vi "OAT State Machine Generate Events for Strings.vi"(1 "Initialize":bool, 2 "Strings":string[](array[string]), 4 "Event":enum16{"Changed"}[](array[ring])) -> (7 "Event Found?":bool[](array[boolean]))   [LabVIEW 2017]
doc: "Detects events for the String objects. When the string is changed, the output is set as TRUE."
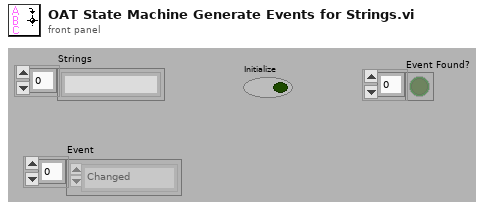
[diagram p1: front panel]
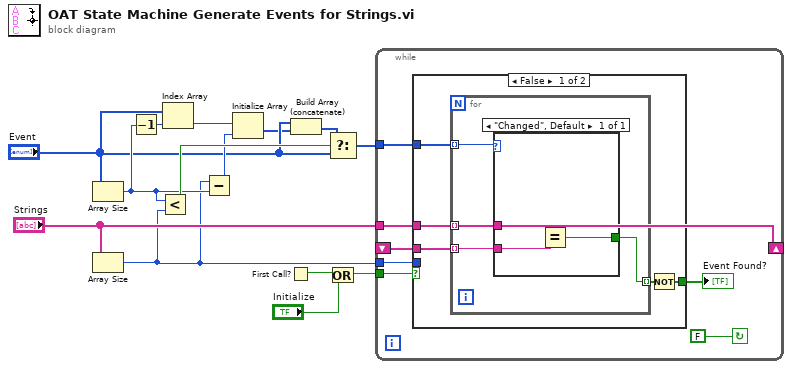
[diagram p0: block diagram]
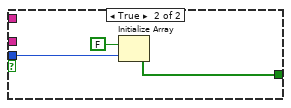
[diagram p2: hidden frame]
diagram:
  n1 = Array Size(array="Event") -> (size(s)=w9:i32)
  n2 = Array Size(array="Strings") -> (size(s)=w4:i32)
  n3 = Decrement(x=w9) -> (x-1=w10:i32)
  n4 = Less?(x=w9, y=w4) -> (x < y?=w11:bool)
  n5 = Index Array(array="Event", index=w10) -> (element=w13:enum16{"Changed"})
  n6 = Subtract(x=w4, y=w9) -> (x-y=w8:i32)
  n7 = Initialize Array(w13, w8) -> (w5:enum16{"Changed"}[])
  n8 = First Call?() -> (First Call?: T/F=w3:bool)
  n9 = Build Array (concatenate)("Event", w5) -> (w7:enum16{"Changed"}[])
  n10 = Select(t=w7, s=w11, f="Event") -> (s? t:f=w12:enum16{"Changed"}[])
  n11 = Or(x=w3, y="Initialize") -> (x .or. y?=w1:bool)
  n12 = while {
    tunnel: w4 -> [w15]
    tunnel: w1 -> [w16]
    tunnel: "Strings" -> [w19]
    shift-left: _ -> [w20]
    shift-right: [w19] -> _
    tunnel: w12 -> [w21]
    stop <- FALSE continue-if-true
    n13 = case shown="False" w16 {
      tunnel: w21 -> [w26 _]
      tunnel: w20 -> [w25 _]
      tunnel: w19 -> [w24 _]
      tunnel: [w22 w34] -> w17
      tunnel: w15 -> [_ w36]
      frame False {
        n14 = for {
          tunnel: w26 -> [w30] mode=indexing
          tunnel: w25 -> [w28] mode=indexing
          tunnel: w24 -> [w29] mode=indexing
          tunnel: [w27] -> w23 mode=indexing
          n15 = case shown="\"Changed\", Default" w30 {
            tunnel: w29 -> [w33]
            tunnel: w28 -> [w32]
            tunnel: [w31] -> w27
            frame "Changed", Default {
              n16 = Equal?(x=w33, y=w32) -> (x = y?=w31:bool)
            }
          }
        }
        n17 = Not(x=w23) -> (.not. x?=w22:bool[])
      }
      frame True {
        n18 = Initialize Array(FALSE, w36) -> (w34:bool[])
      }
    }
    "Event Found?" <- w17
  }
